vi "Read PW Limits.vi"(8 "error in (no error)":errorcluster, 11 "Controller in":refnum<class "Controller.lvclass">) -> (0 "error out":errorcluster, 1 "low pw (us)":dbl, 2 "high pw (us)":dbl, 3 "Controller out":refnum<class "Controller.lvclass">)   [LabVIEW 2020, in "Controller.lvclass"]
uses:
  Controller.lvclass
  Controller.lvclass/Controller.ctl
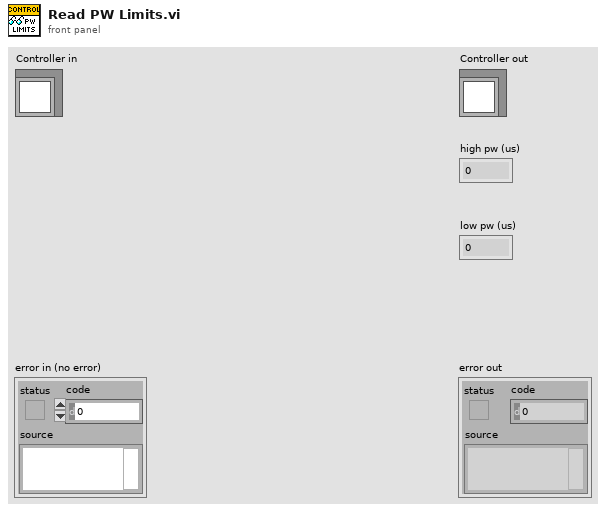
[diagram p1: front panel]
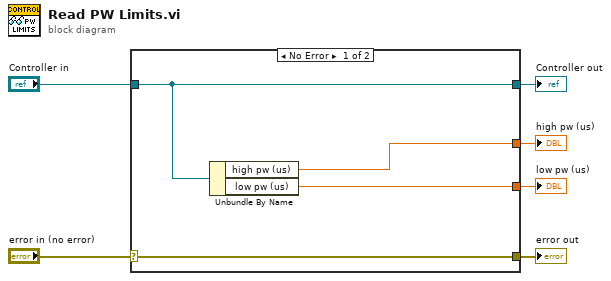
[diagram p0: block diagram]
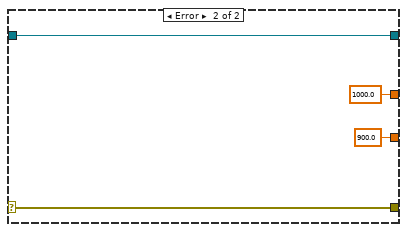
[diagram p2: hidden frame]
diagram:
  n1 = case shown="No Error" "error in (no error)" {
    selector: "error in (no error)" -> [w10 w13]
    tunnel: [w10 w13] -> w5
    tunnel: [w9 w14] -> w3
    tunnel: "Controller in" -> [w9 w14]
    tunnel: [w8 1000.0 ("high pw (us)")] -> w2
    tunnel: [w7 900.0 ("low pw (us)")] -> w1
    frame No Error {
      n2 = Unbundle By Name(w9) -> ("high pw (us)"=w8:dbl, "low pw (us)"=w7:dbl)
    }
    frame Error {
    }
  }
  "error out" <- w5
  "Controller out" <- w3
  "high pw (us)" <- w2
  "low pw (us)" <- w1
